vi "regs.vi"(1 "clear all":bool, 2 "tick":bool, 3 "regs_flags":T2, 4 "input":T3) -> (0 "output":T1)   [LabVIEW 2013]
panel:
  out "dx":T1
  out "cx":T1
  out "bx":T1
  out "ax":T1
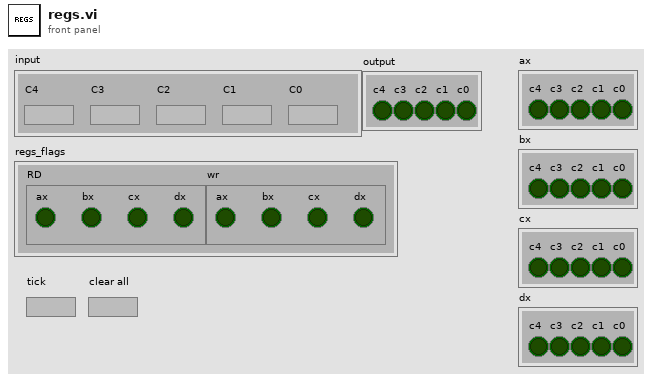
[diagram p1: front panel]
types:
  T1 = cluster{"c4":bool, "c3":bool, "c2":bool, "c1":bool, "c0":bool}
  T2 = cluster{"RD":cluster{"ax":bool, "bx":bool, "cx":bool, "dx":bool}, "wr":cluster{"ax":bool, "bx":bool, "cx":bool, "dx":bool}}
  T3 = cluster{"C4":bool, "C3":bool, "C2":bool, "C1":bool, "C0":bool}
  T4 = cluster{"ax":bool, "bx":bool, "cx":bool, "dx":bool}
  T5 = cluster{"Y4":bool, "Y3":bool, "Y2":bool, "Y1":bool, "Y0":bool}
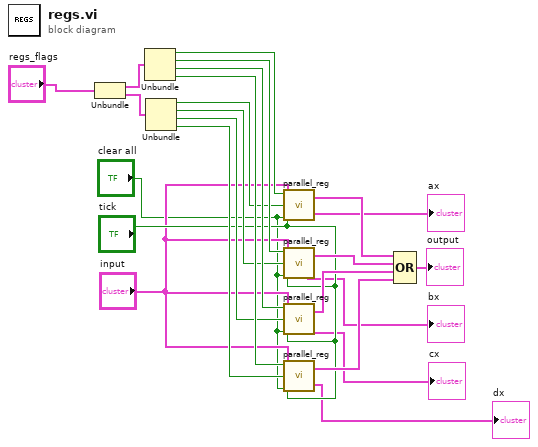
[diagram p0: block diagram]
diagram:
  n1 = Unbundle("regs_flags") -> ("RD"=w18:T4, "wr"=w17:T4)
  n2 = Unbundle(w18) -> ("ax"=w16:bool, "bx"=w13:bool, "cx"=w14:bool, "dx"=w15:bool)
  n3 = Unbundle(w17) -> ("ax"=w12:bool, "bx"=w11:bool, "cx"=w10:bool, "dx"=w9:bool)
  n4 = call "parallel_reg.vi"("RD"=w16, "I"="input", "C"="tick", "R"="clear all", "WR"=w12) -> ("O"=w23:T5, "direct_out"=→"ax":T5)
  n5 = call "parallel_reg.vi"("RD"=w13, "I"="input", "C"="tick", "R"="clear all", "WR"=w11) -> ("O"=w22:T5, "direct_out"=→"bx":T5)
  n6 = call "parallel_reg.vi"("RD"=w14, "I"="input", "C"="tick", "R"="clear all", "WR"=w10) -> ("O"=w20:T5, "direct_out"=→"cx":T5)
  n7 = call "parallel_reg.vi"("RD"=w15, "I"="input", "C"="tick", "R"="clear all", "WR"=w9) -> ("O"=w21:T5, "direct_out"=→"dx":T5)
  n8 = Compound Arithmetic op=OR(w23, w22, w20, w21) -> (→"output":T5)
